vi "Read-Write XYZ movement setup.vi"(6 "Which file? (User profile.ini)":T1=enum."Loaded User profile.ini", 8 "error in":errorcluster, 11 "Function":T2=enum."Load from file") -> (0 "error out":errorcluster)   [LabVIEW 2013]
uses:
  Typedefs/Save-Load enum.ctl
  Typedefs/Which path.ctl
  <vilib>/Utility/config.llb/NI_LVConfig.lvlib
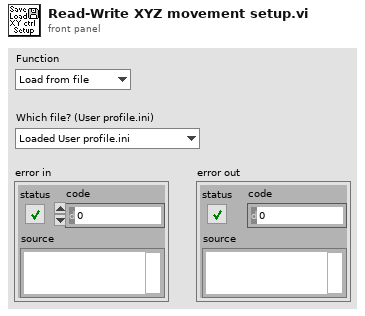
[diagram p1: front panel]
types:
  T1 = typedef "Which path.ctl" = enum16{"Configuration Files", "Calibration Files", "Images", "Setup.ini", "Loaded User profile.ini", "User's-Previous session.ini", "New user profile.ini", "Selected User profile.ini", "User profiles folder", "Power meter scaling.txt", "FOV Cal.ini"}
  T2 = typedef "Save-Load enum.ctl" = enum16{"Save to file", "Load from file", "Compare from file"}
  T3 = typedef "Ini file interface (DBL).ctl" = cluster{"key":string, "Save?":bool, "Default":dbl}[]
  T4 = typedef "Ini file interface (String).ctl" = cluster{"key":string, "Save?":bool, "Default":string}[]
  T5 = typedef "Ini file interface (Boolean).ctl" = cluster{"key":string, "Save?":bool, "Default":bool}[]
  T6 = typedef "NI_LVConfig.lvlib/Config Data RefNum.ctl" = refnum<k1>
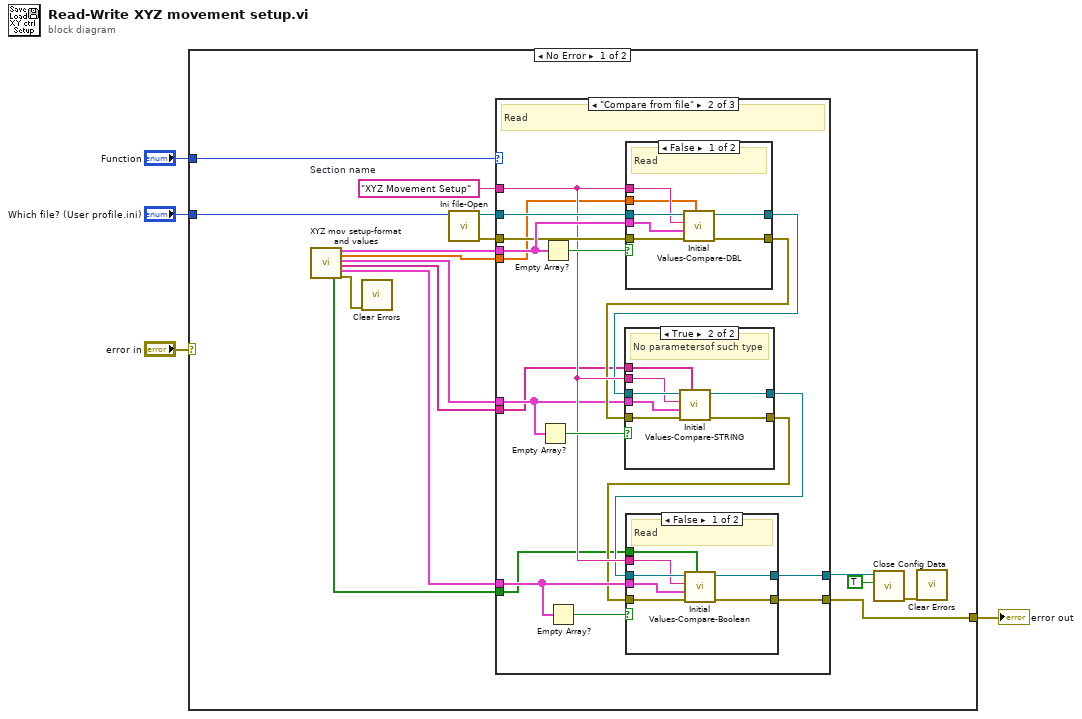
[diagram p0: block diagram]
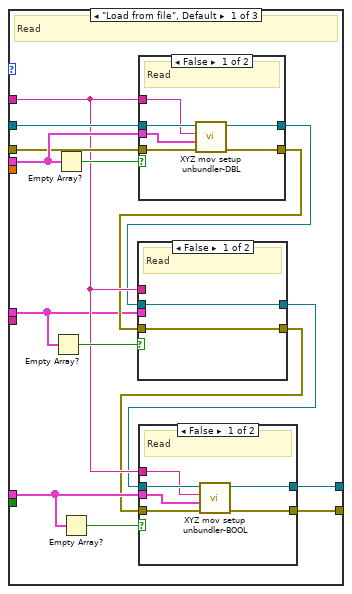
[diagram p2: hidden frame]
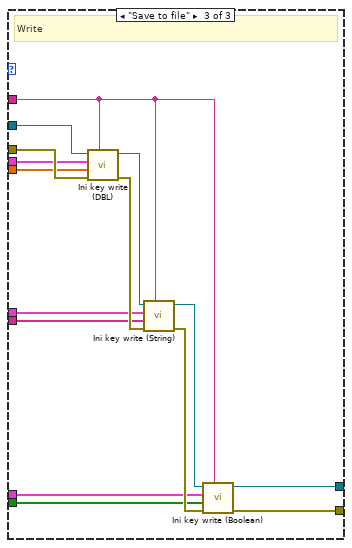
[diagram p9: hidden frame]
diagram:
  n1 = case shown="No Error" "error in" {
    selector: "error in" -> [_ w116]
    tunnel: [w20 w116] -> w4
    tunnel: "Which file? (User profile.ini)" -> [w19 _]
    tunnel: "Function" -> [w18 _]
    frame No Error {
      w11 = "XYZ Movement Setup"  # Section name
      n2 = call "XYZ mov setup-format and values.vi"() -> ("Values.Boolean"=w12:bool[], "Keys setup.DBL"=w17:T3, "Values.DBL"=w16:dbl[], "Keys setup.String"=w15:T4, "Values.Strings"=w14:string[], "Keys setup.Boolean"=w13:T5, "error out"=w5:errorcluster)  [unwired: 13 in]
      n3 = call <vilib>:"Clear Errors.vi"("error in (no error)"=w5) -> ()  [unwired: 6 in, 1 out]
      n4 = call "Ini file-Open.vi"("Which file?"=w19) -> ("error out"=w8:errorcluster, "User profile ini file ref"=w9:T6)  [unwired: 7 in, 2 out]
      n5 = case shown="\"Compare from file\"" w18 {
        tunnel: [w30 w68 w103] -> w20
        tunnel: [w31 w69 w102] -> w7
        tunnel: w8 -> [w32 w70 w114]
        tunnel: w9 -> [w35 w73 w115]
        tunnel: w11 -> [w26 w64 w105]
        tunnel: w17 -> [w34 w72 w112]
        tunnel: w16 -> [_ w58 w113]
        tunnel: w12 -> [_ w57 w104]
        tunnel: w13 -> [w29 w67 w106]
        tunnel: w14 -> [_ w56 w109]
        tunnel: w15 -> [w21 w59 w101]
        frame "Load from file", Default {
          # "Read"
          n6 = Empty Array?(array=w21) -> (empty?=w27:bool)
          n7 = Empty Array?(array=w34) -> (empty?=w33:bool)
          n8 = Empty Array?(array=w29) -> (empty?=w28:bool)
          n9 = case shown="False" w33 {
            tunnel: w35 -> [w51 w55]
            tunnel: [w50 w55] -> w22
            tunnel: [w52 w54] -> w23
            tunnel: w32 -> [w53 w54]
            tunnel: w26 -> [w49 _]
            tunnel: w34 -> [w48 _]
            frame False {
              # "Read"
              n10 = call "XYZ mov setup unbundler-DBL.vi"("error in (no error)"=w53, "Keys Array"=w48, "Section"=w49, "User profile ref"=w51) -> ("error out"=w52:errorcluster, "User profile ref"=w50:T6)  [unwired: 6 in]
            }
            frame True {
              # "No parametersof such type"
            }
          }
          n11 = case shown="False" w27 {
            tunnel: [w36 w39] -> w25
            tunnel: [w37 w38] -> w24
            tunnel: w21 -> [_ _]
            tunnel: w22 -> [w36 w39]
            tunnel: w23 -> [w37 w38]
            tunnel: w26 -> [_ _]
            frame False {
              # "Read"
            }
            frame True {
              # "No parameters of such type"
            }
          }
          n12 = case shown="False" w28 {
            tunnel: [w43 w47] -> w31
            tunnel: [w42 w46] -> w30
            tunnel: w29 -> [w40 _]
            tunnel: w25 -> [w44 w47]
            tunnel: w24 -> [w45 w46]
            tunnel: w26 -> [w41 _]
            frame False {
              # "Read"
              n13 = call "XYZ mov setup unbundler-BOOL.vi"("error in (no error)"=w45, "Keys Array"=w40, "Section name"=w41, "User profile ini file ref"=w44) -> ("error out"=w42:errorcluster, "User profile ini file ref"=w43:T6)  [unwired: 6 in]
            }
            frame True {
              # "No parametersof such type"
            }
          }
        }
        frame "Compare from file" {
          # "Read"
          n14 = Empty Array?(array=w59) -> (empty?=w65:bool)
          n15 = Empty Array?(array=w72) -> (empty?=w71:bool)
          n16 = Empty Array?(array=w67) -> (empty?=w66:bool)
          n17 = case shown="False" w71 {
            tunnel: w73 -> [w98 w100]
            tunnel: [w97 w100] -> w60
            tunnel: [w96 w99] -> w61
            tunnel: w70 -> [w95 w99]
            tunnel: w64 -> [w93 _]
            tunnel: w72 -> [w94 _]
            tunnel: w58 -> [w92 _]
            frame False {
              # "Read"
              n18 = call "Initial Values-Compare-DBL.vi"("Current values"=w92, "error in (no error)"=w95, "Keys Array"=w94, "Section name"=w93, "User profile ini file ref"=w98) -> ("error out"=w96:errorcluster, "User profile ini file ref"=w97:T6)  [unwired: 2 in, 3 out]
            }
            frame True {
              # "No parametersof such type"
            }
          }
          n19 = case shown="True" w65 {
            tunnel: [w75 w81] -> w63
            tunnel: [w74 w79] -> w62
            tunnel: w59 -> [_ w77]
            tunnel: w60 -> [w75 w82]
            tunnel: w61 -> [w74 w80]
            tunnel: w64 -> [_ w78]
            tunnel: w56 -> [_ w76]
            frame False {
              # "Read"
            }
            frame True {
              # "No parametersof such type"
              n20 = call "Initial Values-Compare-STRING.vi"("Current values"=w76, "error in (no error)"=w80, "Keys Array"=w77, "Section name"=w78, "User profile ini file ref"=w82) -> ("error out"=w79:errorcluster, "User profile ini file ref"=w81:T6)  [unwired: 2 in, 3 out]
            }
          }
          n21 = case shown="False" w66 {
            tunnel: [w88 w91] -> w69
            tunnel: [w87 w90] -> w68
            tunnel: w67 -> [w84 _]
            tunnel: w63 -> [w89 w91]
            tunnel: w62 -> [w86 w90]
            tunnel: w64 -> [w85 _]
            tunnel: w57 -> [w83 _]
            frame False {
              # "Read"
              n22 = call "Initial Values-Compare-Boolean.vi"("Current values"=w83, "error in (no error)"=w86, "Keys Array"=w84, "Section name"=w85, "User profile ini file ref"=w89) -> ("error out"=w87:errorcluster, "User profile ini file ref"=w88:T6)  [unwired: 2 in, 3 out]
            }
            frame True {
              # "No parametersof such type"
            }
          }
        }
        frame "Save to file" {
          # "Write"
          n23 = call "Ini key write (DBL).vi"("Section"=w105, "error in (no error)"=w114, "Values (DBL)"=w113, "Ini file interface"=w112, "Ini file refnum in"=w115) -> ("error out"=w110:errorcluster, "Ini file refnum out"=w111:T6)  [unwired: 5 in]
          n24 = call "Ini key write (String).vi"("Section"=w105, "error in (no error)"=w110, "Values (String)"=w109, "Ini file interface"=w101, "Ini file refnum in"=w111) -> ("error out"=w107:errorcluster, "Ini file refnum out"=w108:T6)  [unwired: 5 in]
          n25 = call "Ini key write (Boolean).vi"("Section"=w105, "error in (no error)"=w107, "Values (Boolean)"=w104, "Ini file interface"=w106, "Ini file refnum in"=w108) -> ("error out"=w103:errorcluster, "Ini file refnum out"=w102:T6)  [unwired: 5 in]
        }
      }
      n26 = call <vilib>:"Close Config Data.vi"("write file if changed (T)"=TRUE ("write configuration file? (F)"), "refnum"=w7) -> ("error out"=w6:errorcluster)  [unwired: 8 in, 1 out]
      n27 = call <vilib>:"Clear Errors.vi"("error in (no error)"=w6) -> ()  [unwired: 6 in, 1 out]
    }
    frame Error {
    }
  }
  "error out" <- w4
